vi "Calculate Delivery Time.vi"(8 "error in (no error)":errorcluster, 11 "Pigeon in":refnum<class "Pigeon.lvclass">) -> (0 "error out":errorcluster, 3 "Pigeon out":refnum<class "Pigeon.lvclass">)   [LabVIEW 2019, in "Pigeon.lvclass"]
uses:
  Pigeon.lvclass
  C:/Users/Extensa/Desktop/Fabryka/Fabryka Rozwiazanie/Delivery/Delivery/Delivery.lvclass
  Pigeon.lvclass/Pigeon.ctl
  Delivery/Delivery.lvclass/Delivery.ctl
  Delivery/Delivery.lvclass
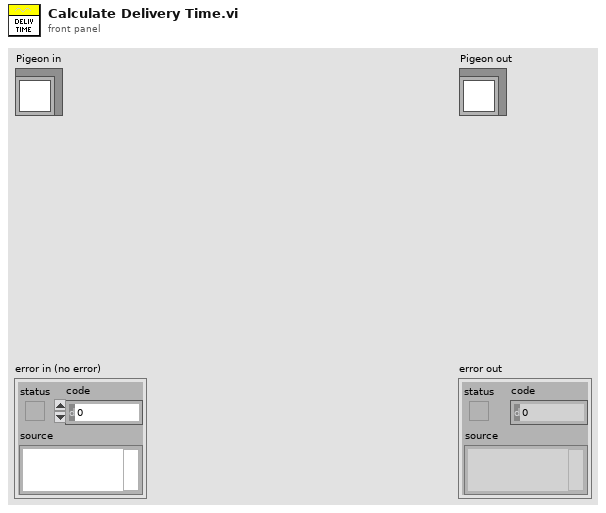
[diagram p1: front panel]
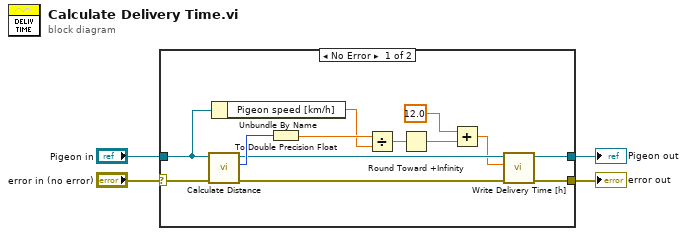
[diagram p0: block diagram]
diagram:
  n1 = case shown="No Error" "error in (no error)" {
    selector: "error in (no error)" -> [w17 w19]
    tunnel: [w5 w19] -> w3
    tunnel: [w6 w18] -> w1
    tunnel: "Pigeon in" -> [w16 w18]
    frame No Error {
      n2 = call "Calculate Distance.vi"("error in (no error)"=w17, "Pigeon in"=w16) -> ("error out"=w9:errorcluster, "Distance [km]"=w15:i32, "Pigeon out"=w8:refnum<class "Pigeon.lvclass">)  [unwired: 7 in]
      n3 = Unbundle By Name(w16) -> ("Pigeon speed [km/h]"=w13:dbl)
      n4 = To Double Precision Float(number=w15) -> (double precision float=w14:dbl)
      n5 = Divide(x=w14, y=w13) -> (x/y=w12:dbl)
      n6 = Round Toward +Infinity(x=w12) -> (ceil(x): smallest int >= x=w11:dbl)
      n7 = Add(x=12.0, y=w11) -> (x+y=w7:dbl)
      n8 = call "Write Delivery Time [h].vi"("error in (no error)"=w9, "Delivery Time [h]"=w7, "Delivery in"=w8) -> ("error out"=w5:errorcluster, "Delivery out"=w6:refnum<class "Pigeon.lvclass">)  [unwired: 7 in]
    }
    frame Error {
    }
  }
  "error out" <- w3
  "Pigeon out" <- w1
